vi "Intake process.vi"   [LabVIEW 2013]
uses:
  Intake Global.vi
types:
  T1 = cluster{"Gripper":dbl, "Upper Jaw":dbl, "Ball Limit Switch":bool, "Upper Limit Switch":bool, "Lower Limit Switch ":bool}
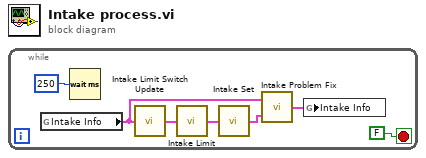
[diagram p0: block diagram]
diagram:
  n1 = while {
    stop <- FALSE stop-if-true
    n2 = global read "Intake Global.vi" "Intake Info"() -> (w2:T1)
    n3 = Wait (ms)(milliseconds to wait=u32 250) -> ()  [unwired: 1 out]
    n4 = call "Intake Limit Switch Update.vi"("Intake Info In"=w2) -> ("Intake Info Out"=w5:T1)
    n5 = call "Intake Limit.vi"("Intake Info In"=w5) -> ("Intake Info Out"=w4:T1)
    n6 = call "Intake Set.vi"("Intake Info In"=w4) -> ("Intake Info Out"=w3:T1)
    n7 = call "Intake Problem Fix.vi"("Intake Info Modified"=w3, "Intake Info Original"=w2) -> ("Intake Info Fixed"=w1:T1)
    n8 = global write "Intake Global.vi" "Intake Info"(w1) -> ()
  }
